vi "Wait for SRQ.vi"(0 "VISA resource name":refnum<visa-resource-name>, 4 "SRQ Enable Command":string, 5 "error in (no error)":errorcluster, 8 "Timeout (25000 ms)":u32=25000) -> (14 "VISA resource name out":refnum<visa-resource-name>, 19 "error out":errorcluster)   [LabVIEW 2016, in "Keithley 2000.lvlib"]
doc: "This VI waits for a service request from the instrument. The service request must be enabled on the instrument prior to calling this VI."
uses:
  Keithley 2000.lvlib
  <vilib>/Instr/_visa.llb/Select Event Type.ctl
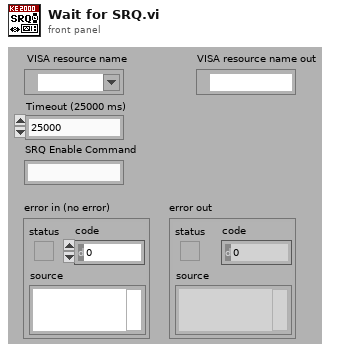
[diagram p1: front panel]
types:
  T1 = typedef "Select Event Type.ctl" = u32
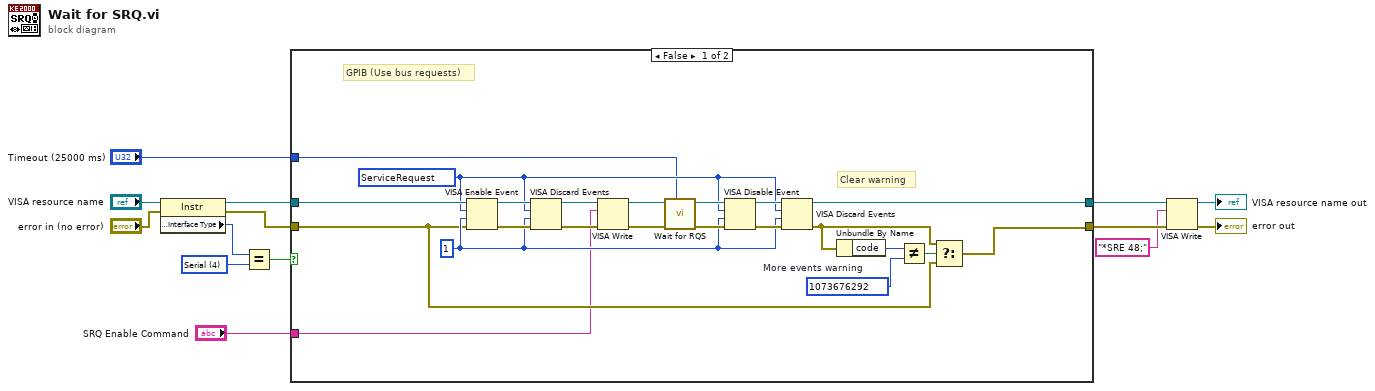
[diagram p0: block diagram]
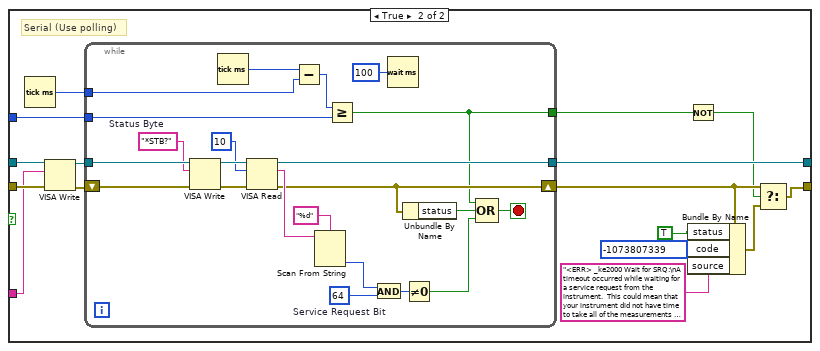
[diagram p2: hidden frame]
diagram:
  w9 = u16 4 items=["GPIB"=1, "VXI"=2, "GPIB-VXI"=3, "Serial"=4, "PXI"=5, "TCPIP"=6, "USB"=7] ("Interface Information:Interface Type")
  n1 = property class="Instr"(reference="VISA resource name", error in="error in (no error)") -> (reference out=w7:refnum<visa-resource-name>, error out=w11:errorcluster, "Interface Information:Interface Type"=w10:u16)
  n2 = Equal?(x=w10, y=w9) -> (x = y?=w8:bool)
  n3 = case shown="False" w8 {
    tunnel: w7 -> [w34 w39]
    tunnel: "Timeout (25000 ms)" -> [w27 w52]
    tunnel: [w26 w44] -> w3
    tunnel: [w21 w51] -> w2
    tunnel: w11 -> [w20 w38]
    tunnel: "SRQ Enable Command" -> [w15 w37]
    frame False {
      w24 = 1073676292  # More events warning
      w29 = u16 1 ("mechanism (1:  VI_QUEUE)")
      w28 = T1 1073684491 items=["ServiceRequest"=1073684491, "Trigger"=3221168138, "Clear"=1073684493, "VXI-Signal"=1073684512, "VXI/VME-Interrupt"=3221168161, "VXI/VME-Sysfail"=1073684509, "VXI/VME-Sysreset"=1073684510, "GPIB-CIC"=1073684498, "GPIB-Talk"=1073684499, "GPIB-Listen"=1073684500, "PXI-Interrupt"=1073684514, "Serial-Break"=1073684515, "Serial-TermChar"=1073684516, "Serial-CTS"=1073684521, "Serial-DSR"=1073684522, "Serial-DCD"=1073684524, "Serial-RI"=1073684526, "Serial-Character"=1073684533, "USB-Interrupt"=1073684535, "AllEnabled"=1073709055] ("Event Type")
      # "GPIB (Use bus requests)"
      # "Clear warning"
      n4 = VISA Enable Event(8:w20, 9:w29, 10:w28, 11:w34) -> (0:w35:errorcluster, 3:w36:refnum<visa-resource-name>)
      n5 = VISA Discard Events(8:w35, 9:w29, 10:w28, 11:w36) -> (0:w18:errorcluster, 3:w19:refnum<visa-resource-name>)
      n6 = VISA Write(VISA resource name=w19, write buffer=w15, error in (no error)=w18) -> (VISA resource name out=w17:refnum<visa-resource-name>, error out=w16:errorcluster)  [unwired: 1 out]
      n7 = call <vilib>:"Wait for RQS.VI"("timeout (25000 ms)"=w27, "error in (no error)"=w16, "VISA resource name"=w17) -> ("error out"=w31:errorcluster, "VISA resource name out"=w33:refnum<visa-resource-name>)  [unwired: 6 in, 1 out]
      n8 = VISA Disable Event(8:w31, 9:w29, 10:w28, 11:w33) -> (0:w30:errorcluster, 3:w32:refnum<visa-resource-name>)
      n9 = VISA Discard Events(8:w30, 9:w29, 10:w28, 11:w32) -> (0:w22:errorcluster, 3:w26:refnum<visa-resource-name>)
      n10 = Unbundle By Name(w22) -> ("code"=w25:i32)
      n11 = Not Equal?(x=w25, y=w24) -> (x != y?=w23:bool)
      n12 = Select(t=w22, s=w23, f=w20) -> (s? t:f=w21:errorcluster)
    }
    frame True {
      # "Serial (Use polling)"
      n13 = Tick Count (ms)() -> (millisecond timer value=w45:u32)
      n14 = VISA Write(VISA resource name=w39, write buffer=w37, error in (no error)=w38) -> (VISA resource name out=w41:refnum<visa-resource-name>, error out=w40:errorcluster)  [unwired: 1 out]
      n15 = while {
        shift-right: [w55] -> w50
        shift-left: w40 -> [w65]
        tunnel: w52 -> [w68]
        tunnel: w41 -> [w66]
        tunnel: w45 -> [w70]
        tunnel: [w62] -> w44
        tunnel: [w53] -> w43
        stop <- w73 stop-if-true
        w60 = "*STB?"  # Status Byte
        w61 = 64  # Service Request Bit
        n16 = VISA Write(VISA resource name=w66, write buffer=w60, error in (no error)=w65) -> (VISA resource name out=w63:refnum<visa-resource-name>, error out=w64:errorcluster)  [unwired: 1 out]
        n17 = Tick Count (ms)() -> (millisecond timer value=w71:u32)
        n18 = VISA Read(VISA resource name=w63, byte count=u32 10, error in (no error)=w64) -> (VISA resource name out=w62:refnum<visa-resource-name>, read buffer=w58:string, error out=w55:errorcluster)  [unwired: 1 out]
        n19 = Subtract(x=w71, y=w70) -> (x-y=w69:u32)
        n20 = Scan From String(format string="%d", input string=w58) -> (output 1=w56:i32)  [unwired: 3 in, 3 out]
        n21 = Greater Or Equal?(x=w69, y=w68) -> (x >= y?=w53:bool)
        n22 = And(x=w56, y=w61) -> (x .and. y?=w74:i32)
        n23 = Wait (ms)(milliseconds to wait=u32 100) -> ()  [unwired: 1 out]
        n24 = Unbundle By Name(w55) -> ("status"=w54:bool)
        n25 = Not Equal To 0?(x=w74) -> (x != 0?=w72:bool)
        n26 = Compound Arithmetic op=OR(w53, w54, w72) -> (w73:bool)
      }
      n27 = Not(x=w43) -> (.not. x?=w42:bool)
      n28 = Bundle By Name(cluster=w50, "status"=TRUE, "code"=-1073807339, "source"="<ERR> _ke2000 Wait for SRQ:\nA timeout occurred while waiting for a service request from the instrument.  This could mean that your instrument did not have time to take all of the measurements or that an error occurred previously.") -> (w47:errorcluster)
      n29 = Select(t=w50, s=w42, f=w47) -> (s? t:f=w51:errorcluster)
    }
  }
  n30 = VISA Write(VISA resource name=w3, write buffer="*SRE 48;", error in (no error)=w2) -> (VISA resource name out=→"VISA resource name out":refnum<visa-resource-name>, error out=→"error out":errorcluster)  [unwired: 1 out]
